vi "Performance.vi"() -> ()   [LabVIEW 2013]
uses:
  <vilib>/Heliosphere Research LLC/Advanced Plotting Toolkit/api_figure/TicksProperties.ctl
  <vilib>/Heliosphere Research LLC/Advanced Plotting Toolkit/properties/Text.ctl
  <vilib>/Heliosphere Research LLC/Advanced Plotting Toolkit/typedefs/PlotColor.ctl
  <vilib>/Heliosphere Research LLC/Advanced Plotting Toolkit/properties/Text_FontSize.ctl
  <vilib>/Heliosphere Research LLC/Advanced Plotting Toolkit/properties/Text_FontStyle.ctl
  <vilib>/Heliosphere Research LLC/Advanced Plotting Toolkit/api_core/NewPlotProperties.ctl
  <vilib>/Utility/sysdir.llb/System Directory Type.ctl
  <vilib>/Heliosphere Research LLC/Advanced Plotting Toolkit/Advanced Plotting Toolkit.lvlib
panel:
  out "Picture":picture
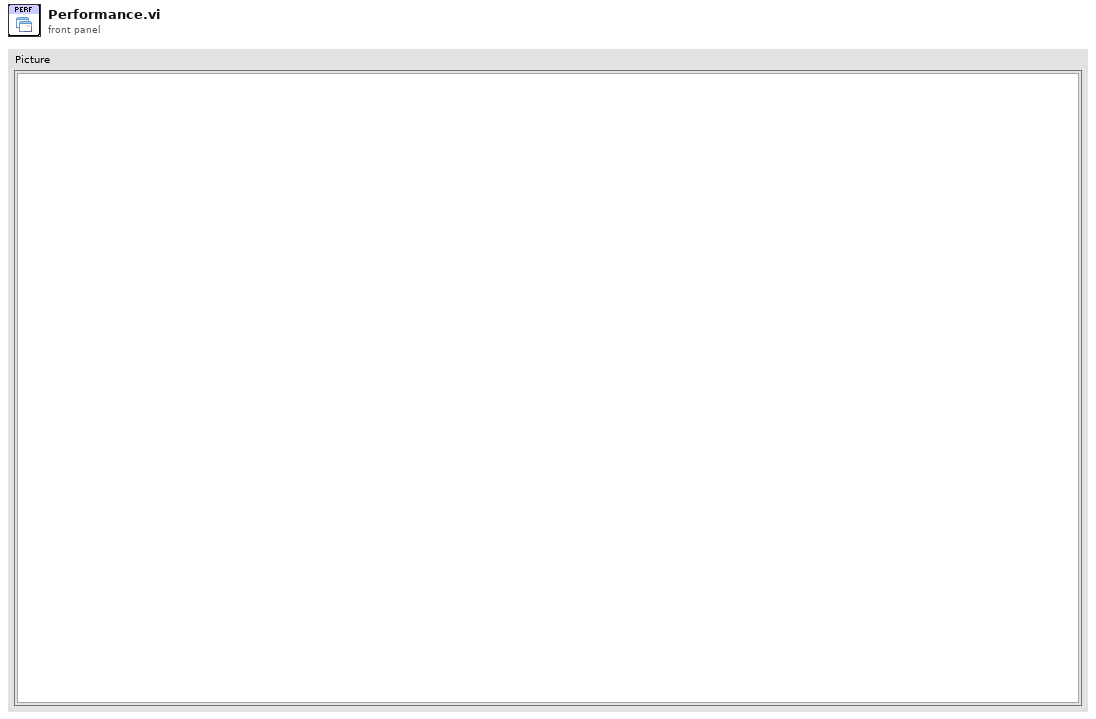
[diagram p1: front panel]
types:
  T1 = typedef "System Directory Type.ctl" = i32
  T2 = typedef "Advanced Plotting Toolkit.lvlib/NewPlotProperties.ctl" = cluster{"Background Color":T3, "Axis Background":T3, "Left Margin":dbl, "Right Margin":dbl, "Bottom Margin":dbl, "Top Margin":dbl, "Aspect Ratio":dbl}
  T3 = typedef "Advanced Plotting Toolkit.lvlib/PlotColor.ctl" = u32
  T4 = typedef "Advanced Plotting Toolkit.lvlib/TicksProperties.ctl" = cluster{"Text":T5}
  T5 = typedef "Advanced Plotting Toolkit.lvlib/Text.ctl" = cluster{"Color":T3, "Background Color":T3, "Font Size (points)":T6, "Font Style":T7, "Rotation Angle":dbl}
  T6 = typedef "Advanced Plotting Toolkit.lvlib/Text_FontSize.ctl" = i32
  T7 = typedef "Advanced Plotting Toolkit.lvlib/Text_FontStyle.ctl" = enum16{"Automatic", "Normal", "Italic", "Bold"}
  T8 = typedef "Advanced Plotting Toolkit.lvlib/PlotID.ctl" = i32
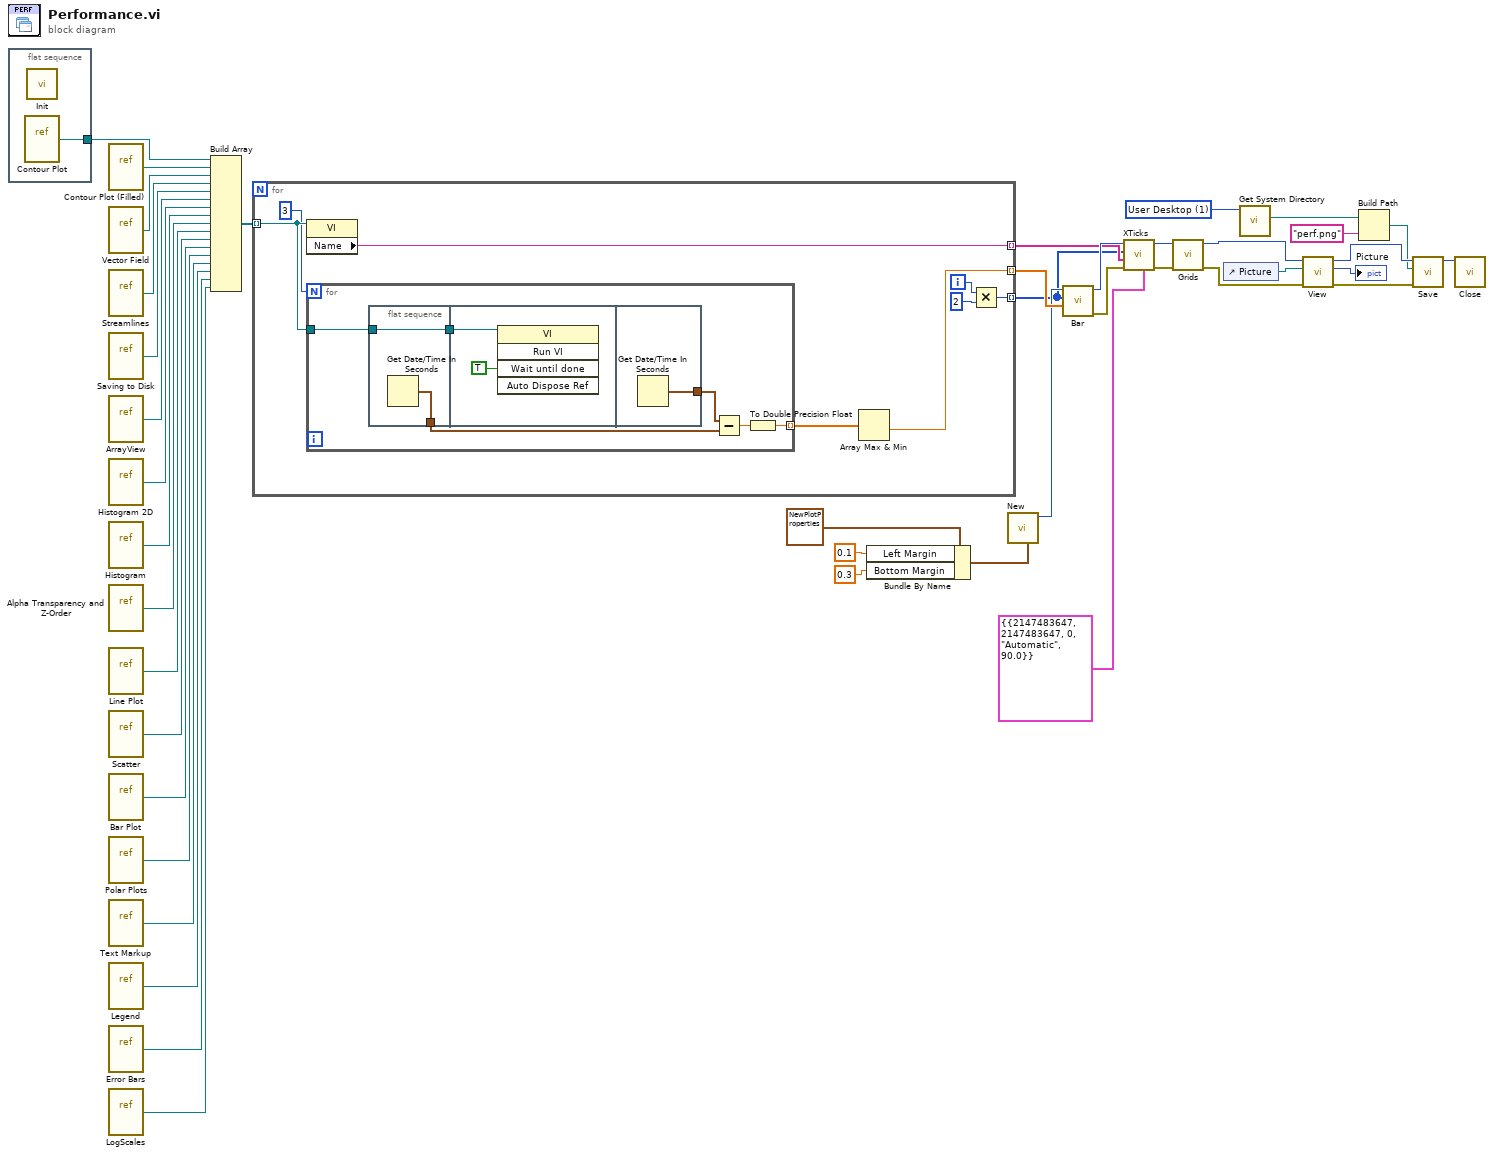
[diagram p0: block diagram]
diagram:
  w4 = T1 1 items=["User Home"=0, "User Desktop"=1, "User Documents"=2, "User Application Data"=3, "User Preferences"=4, "User Temporary"=5, "Public Documents"=6, "Public Application Data"=7, "Public Preferences"=8, "Public Cache"=13, "System Core Libraries"=9, "System Installed Libraries"=10, "Application Files"=11, "Boot Volume Root"=12] ("system directory type")
  n1 = flat-sequence {
    tunnel: [w43] -> w26
    frame #0 {
      n2 = vi-ref "Contour Plot.vi"() -> (w43:refnum<vi>)
      n3 = call <vilib>:"Init.vi"() -> ()  [unwired: 11 in, 1 out]
    }
  }
  n4 = vi-ref "Contour Plot (Filled).vi"() -> (w42:refnum<vi>)
  n5 = vi-ref "Vector Field.vi"() -> (w41:refnum<vi>)
  n6 = vi-ref "Streamlines.vi"() -> (w40:refnum<vi>)
  n7 = vi-ref "Saving to Disk.vi"() -> (w27:refnum<vi>)
  n8 = vi-ref "ArrayView.vi"() -> (w39:refnum<vi>)
  n9 = vi-ref "Histogram 2D.vi"() -> (w38:refnum<vi>)
  n10 = vi-ref "Histogram.vi"() -> (w37:refnum<vi>)
  n11 = vi-ref "Alpha Transparency and Z-Order.vi"() -> (w36:refnum<vi>)
  n12 = vi-ref "Line Plot.vi"() -> (w35:refnum<vi>)
  n13 = vi-ref "Scatter.vi"() -> (w34:refnum<vi>)
  n14 = vi-ref "Bar Plot.vi"() -> (w33:refnum<vi>)
  n15 = vi-ref "Polar Plots.vi"() -> (w32:refnum<vi>)
  n16 = vi-ref "Text Markup.vi"() -> (w31:refnum<vi>)
  n17 = vi-ref "Legend.vi"() -> (w30:refnum<vi>)
  n18 = vi-ref "Error Bars.vi"() -> (w29:refnum<vi>)
  n19 = vi-ref "LogScales.vi"() -> (w28:refnum<vi>)
  n20 = Build Array(w26, w42, w41, w40, w27, w39, w38, w37, w36, w35, w34, w33, w32, w31, w30, w29, w28) -> (w25:refnum<vi>[])
  n21 = for {
    tunnel: w25 -> [w51] mode=indexing
    tunnel: [w50] -> w21 mode=indexing
    tunnel: [w48] -> w24 mode=indexing
    tunnel: [w45] -> w19 mode=indexing
    i -> [w46]
    n22 = property class="VI"(reference=w51) -> ("Name"=w50:string)  [unwired: 1 in, 2 out]
    n23 = for {
      N: 3 -> [_]
      tunnel: [w53] -> w49 mode=indexing
      tunnel: w51 -> [w52]
      n24 = flat-sequence {
        tunnel: w52 -> [w59]
        tunnel: [w59] -> w57
        tunnel: [w58] -> w56
        tunnel: w57 -> [w60]
        tunnel: [w62] -> w55
        frame #0 {
          n25 = Get Date/Time In Seconds() -> (seconds since 1Jan1904=w58:timestamp)
        }
        frame #1 {
          n26 = invoke class="VI" method="Run VI"(reference=w60, "Wait until done"=TRUE ("Wait Until Done")) -> ()  [unwired: 3 in, 5 out]
        }
        frame #2 {
          n27 = Get Date/Time In Seconds() -> (seconds since 1Jan1904=w62:timestamp)
        }
      }
      n28 = Subtract(x=w55, y=w56) -> (x-y=w54:dbl)
      n29 = To Double Precision Float(number=w54) -> (double precision float=w53:dbl)
    }
    n30 = Array Max & Min(array=w49) -> (min value=w48:dbl)  [unwired: 3 out]
    n31 = Multiply(x=w46, y=2) -> (x*y=w45:i32)
  }
  n32 = Bundle By Name(cluster=T2 {"Background Color"=2147483647, "Axis Background"=2147483647, "Left Margin"=nan, "Right Margin"=nan, "Bottom Margin"=nan, "Top Margin"=nan, "Aspect Ratio"=nan} ("New Plot Properties"), "Left Margin"=0.1, "Bottom Margin"=0.3 ("Top Margin")) -> (w14:T2)
  n33 = call <vilib>:"New.vi"("Properties"=w14) -> ("Plot ID"=w22:T8)  [unwired: 9 in, 1 out]
  n34 = call <vilib>:"Bar.vi"("Bar Lengths"=w24, "X Coordinates"=w19, "Plot ID"=w22) -> ("error out"=w20:errorcluster, "Plot ID Out"=w23:T8)  [unwired: 7 in]
  n35 = call <vilib>:"XTicks.vi"("Properties"=T4 {"Text"={"Color"=2147483647, "Background Color"=2147483647, "Font Size (points)"=0, "Font Style"=enum."Automatic", "Rotation Angle"=90.0}} ("Tick Properties"), "error in (no error)"=w20, "Tick Labels"=w21, "Tick Locations"=w19, "Plot ID"=w23) -> ("error out"=w9:errorcluster, "Plot ID Out"=w11:T8)  [unwired: 5 in]
  n36 = call <vilib>:"Grids.vi"("error in (no error)"=w9, "Plot ID"=w11) -> ("error out"=w8:errorcluster, "Plot ID Out"=w10:T8)  [unwired: 8 in]
  n37 = control-ref of="Picture"() -> (w17:refnum<vi>)
  n38 = call <vilib>:"Get System Directory.vi"("system directory type"=w4) -> ("system directory"=w3:path)  [unwired: 10 in]
  n39 = call <vilib>:"View.vi"("error in (no error)"=w8, "Ref for Sizing"=w17, "Plot ID"=w10) -> ("error out"=w5:errorcluster, "Picture"=→"Picture":picture, "Plot ID Out"=w7:T8)  [unwired: 6 in]
  n40 = Build Path(base path=w3, name or relative path="perf.png") -> (appended path=w1:path)
  n41 = call <vilib>:"Save.vi"("error in (no error)"=w5, "Path"=w1, "Plot ID In"=w7) -> ("Plot ID Out"=w6:T8)  [unwired: 7 in, 1 out]
  n42 = call <vilib>:"Close.vi"("Plot ID"=w6) -> ()  [unwired: 11 in]
